vi "Abyss-watcher_love-edition.vi"(8 "stop":bool) -> (1 "moving?":bool, 2 "hot-map":i16[][](graph), 3 "varience":dbl[](graph))   [LabVIEW 2021]
uses:
  <vilib>/userdefined/High Color/IMAQdx.ctl
  382ecd2c-2874-4518-af08-13692d44ced6.vi
  <vilib>/Analysis/baseanly.llb/Mean (DBL).vi
  <vilib>/Comparison/Less/Less Functor/Less Functor.lvclass
  <vilib>/vision/driver/NI_Vision_Acquisition_Software.lvlib
  <vilib>/Analysis/NI_AALBase.lvlib
panel:
  out "greyscale Graph":i16[][](graph)
  in  "threshold":dbl=7.5
  out "varience":dbl
  out "mean":dbl format="%0.2f"
  out "?":T1(plugin-control)
  out "average\n Graph":dbl[](graph)
  in  "y length":i32=400
  in  "roiy":i32=250
  in  "x length":i32=300
  in  "roix":i32=825
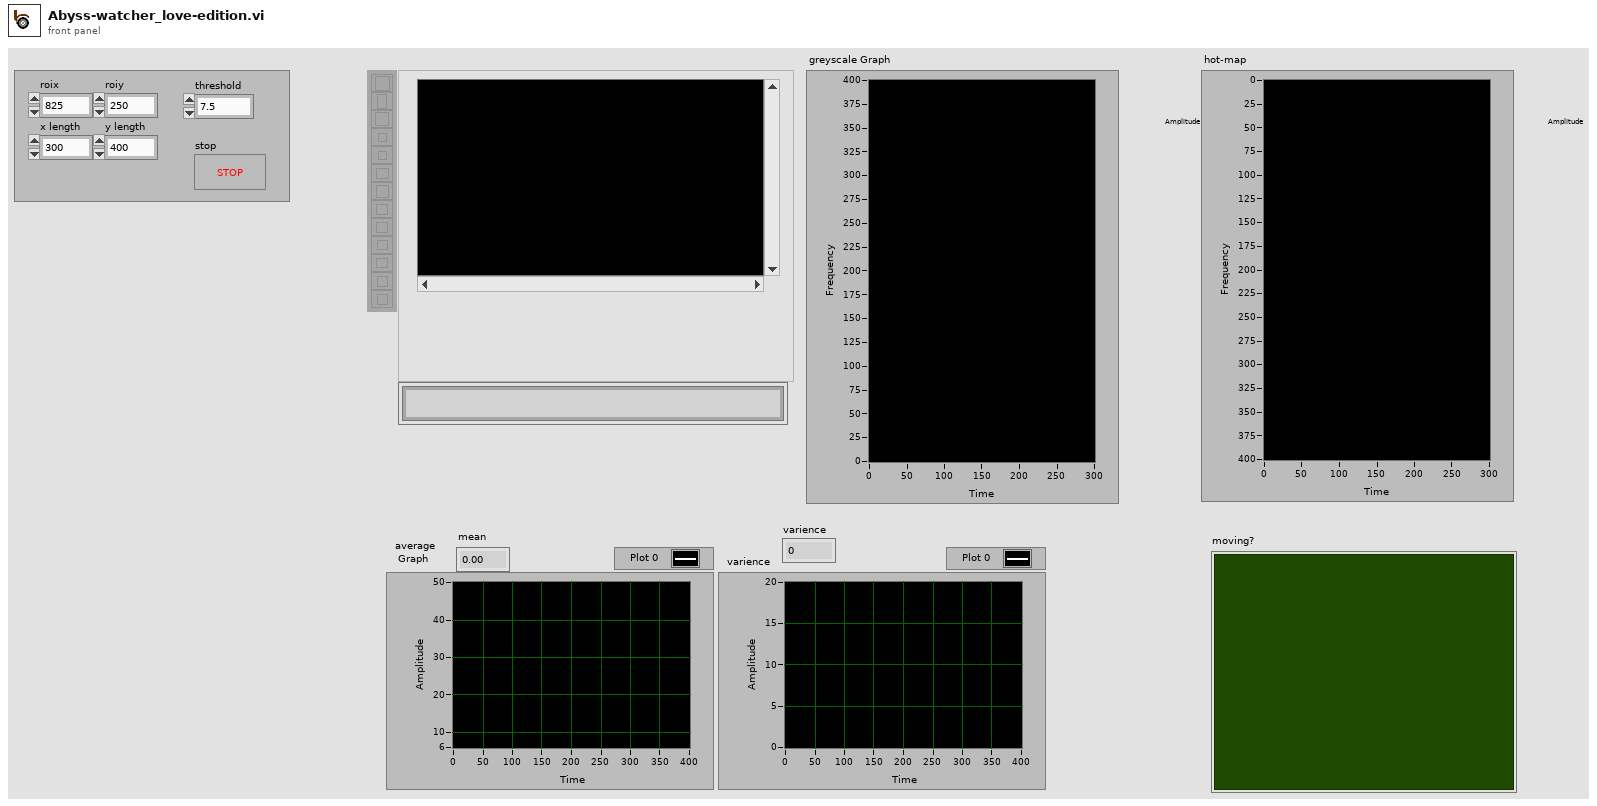
[diagram p1: front panel]
types:
  T1 = typedef "IMAQ Image.ctl" = refnum<image>
  T2 = typedef "Image Type" = u32
  T3 = typedef "IMAQdx.ctl" = refnum<k21>
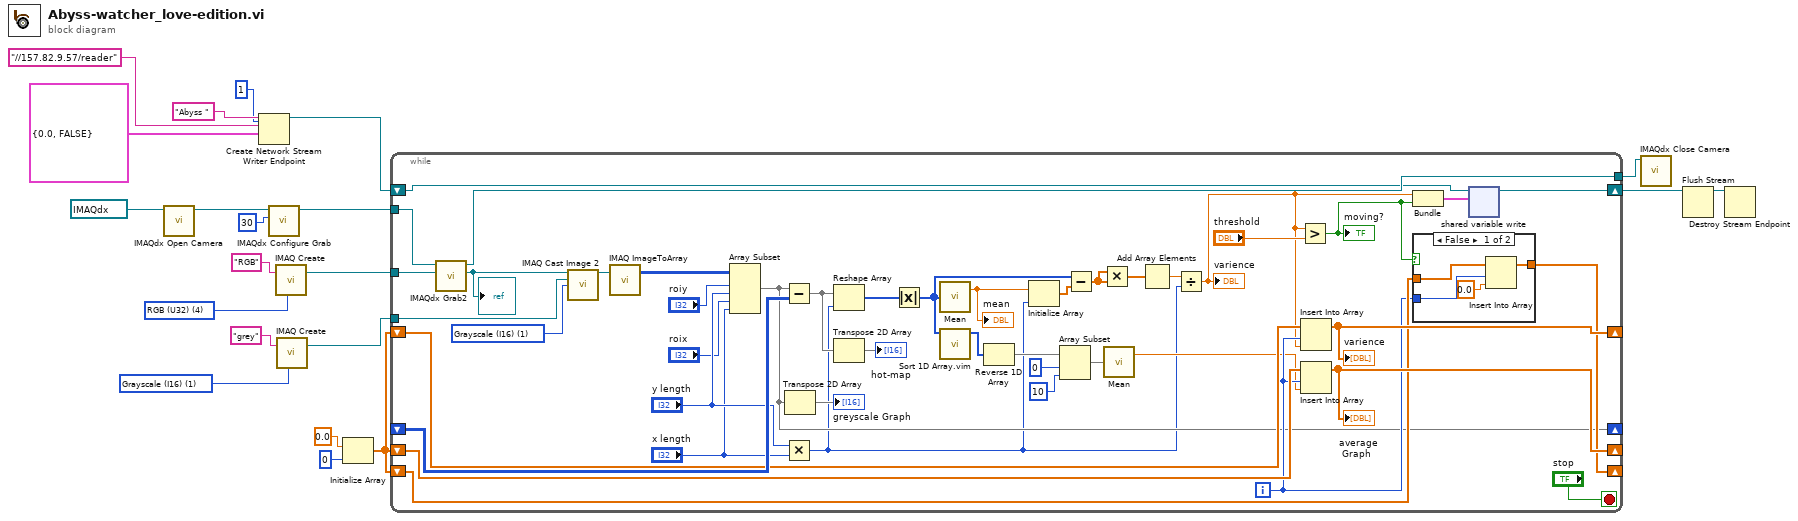
[diagram p0: block diagram]
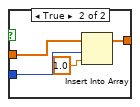
[diagram p2: hidden frame]
diagram:
  w14 = T2 1 items=["Grayscale (U8)", "Grayscale (I16)", "Grayscale (SGL)", "Complex (CSG)", "RGB (U32)", "HSL (U32)", "RGB (U64)", "Grayscale (U16)"] ("Image Type")
  w15 = T2 4 items=["Grayscale (U8)", "Grayscale (I16)", "Grayscale (SGL)", "Complex (CSG)", "RGB (U32)", "HSL (U32)", "RGB (U64)", "Grayscale (U16)"] ("Image Type")
  n1 = call <vilib>:"IMAQdx Open Camera.vi"("Session In"=T3 "cam2") -> ("Session Out"=w19:T3)  [unwired: 9 in, 1 out]
  n2 = Create Network Stream Writer Endpoint(7:1 ("writer buffer size"), 9:cluster{dbl, bool} {0.0, FALSE}, 10:"//157.82.9.57/reader" ("reader url"), 11:"Abyss " ("writer name")) -> (3:w6:refnum<k21>)  [unwired: 3 in, 1 out]
  n3 = call <vilib>:"IMAQdx Configure Grab.vi"("Number of Buffers"=u32 30, "Session In"=w19) -> ("Session Out"=w17:T3)  [unwired: 8 in, 1 out]
  n4 = call "IMAQ Create"("Image Name"="RGB", "Image Type"=w15) -> ("New Image"=w16:T1)  [unwired: 3 in, 1 out]
  n5 = call "IMAQ Create"("Image Name"="grey", "Image Type"=w14) -> ("New Image"=w13:T1)  [unwired: 3 in, 1 out]
  n6 = Initialize Array(0.0 ("element"), 0 ("dimension size")) -> (w8:dbl[])
  n7 = while {
    tunnel: w17 -> [w66]
    tunnel: w16 -> [w65]
    tunnel: w13 -> [w64]
    tunnel: [w63] -> w12
    shift-right: [w27] -> _
    shift-left: _ -> [w62]
    shift-right: [w58] -> _
    shift-left: w8 -> [w61]
    shift-right: [w49] -> _
    shift-left: w8 -> [w50]
    shift-right: [w45] -> _
    shift-left: w8 -> [w47]
    shift-right: [w32] -> w5
    shift-left: w6 -> [w33]
    i -> [w46]
    stop <- "stop" stop-if-true
    w60 = T2 1 items=["Grayscale (U8)", "Grayscale (I16)", "Grayscale (SGL)", "Complex (CSG)", "RGB (U32)", "HSL (U32)", "RGB (U64)", "Grayscale (U16)"] ("Image Type")
    n8 = call <vilib>:"IMAQdx Grab2.vi"("Image In"=w65, "Session In"=w66) -> ("Image Out"=w35:T1, "Session Out"=w63:T3)  [unwired: 6 in, 2 out]
    "?" <- w35
    n9 = call "IMAQ Cast Image 2"("Image Src"=w35, "Image Dst"=w64, "Image Type"=w60) -> ("Image Dst Out"=w59:T1)  [unwired: 11 in, 1 out]
    n10 = call "IMAQ ImageToArray"("Image"=w59) -> ("Image Pixels (I16)"=w57:i16[][])  [unwired: 3 in, 4 out]
    n11 = Array Subset(array=w57, index (row)="roiy", length (row)="y length", index (col)="roix", length (col)="x length") -> (w27:i16[][])
    n12 = Subtract(x=w27, y=w62) -> (x-y=w44:i16[][])
    n13 = Multiply(x="y length", y="x length") -> (x*y=w26:i32)
    n14 = Transpose 2D Array(2D array=w27) -> (transposed array=→"greyscale Graph":i16[][])
    n15 = Reshape Array(w44, w26) -> (w56:i16[])
    n16 = Transpose 2D Array(2D array=w44) -> (transposed array=→"hot-map":i16[][])
    n17 = Absolute Value(x=w56) -> (abs(x)=w42:i16[])
    n18 = call-poly <vilib>:"Mean.vi"("X"=w42) -> ("mean"=w54:dbl)  [unwired: 1 out]
    "mean" <- w54
    n19 = call "Sort 1D Array.vim"("unsorted array"=w42) -> ("sorted array"=w40:i16[])  [unwired: 10 in]
    n20 = Reverse 1D Array(array=w40) -> (reversed array=w39:i16[])
    n21 = Initialize Array(w54, w26) -> (w53:dbl[])
    n22 = Array Subset(array=w39, index=0, length=10) -> (w37:i16[])
    n23 = Subtract(x=w42, y=w53) -> (x-y=w52:dbl[])
    n24 = Multiply(x=w52, y=w52) -> (x*y=w51:dbl[])
    n25 = call-poly <vilib>:"Mean.vi"("X"=w37) -> ("mean"=w36:dbl)  [unwired: 1 out]
    n26 = Add Array Elements(numeric array=w51) -> (sum=w55:dbl)
    n27 = Divide(x=w55, y=w26) -> (x/y=w31:dbl)
    "varience" <- w31
    n28 = Greater?(x=w31, y="threshold") -> (0:w30:bool)
    "moving?" <- w30
    n29 = Insert Into Array(array=w50, index=w46, new element=w31) -> (w49:dbl[])
    "varience" <- w49
    n30 = Insert Into Array(array=w61, index=w46, new element=w36) -> (w58:dbl[])
    "average\n Graph" <- w58
    n31 = Bundle(w31, w30) -> (w29:cluster{dbl, bool})  [unwired: 1 in]
    n32 = case shown="False" w30 {
      tunnel: [w67 w74] -> w45
      tunnel: w47 -> [w70 w73]
      tunnel: w46 -> [w69 w72]
      frame False {
        n33 = Insert Into Array(array=w70, index=w69, new element=0.0 ("new element/subarray")) -> (w67:dbl[])
      }
      frame True {
        n34 = Insert Into Array(array=w73, index=w72, new element=1.0 ("new element/subarray")) -> (w74:dbl[])
      }
    }
    n35 = shared-variable-write(w33, w29) -> (w32:refnum<k21>)  [unwired: 2 in, 2 out]
  }
  n36 = call <vilib>:"IMAQdx Close Camera.vi"("Session In"=w12) -> ()  [unwired: 10 in, 1 out]
  n37 = Flush Stream(11:w5) -> (3:w4:refnum<k21>)  [unwired: 3 in, 2 out]
  n38 = Destroy Stream Endpoint(11:w4) -> ()  [unwired: 1 in, 1 out]
